vi "oa_SCL Min Max X.vi"(1 "scaled xy data":cluster{"x":i16, "y":i16}[](array[cluster])) -> (0 "min max data":cluster{"x":i16, "min":i16, "max":i16}[](array[cluster]))   [LabVIEW 2017]
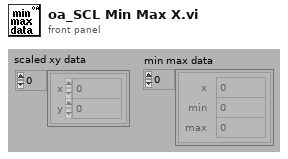
[diagram p1: front panel]
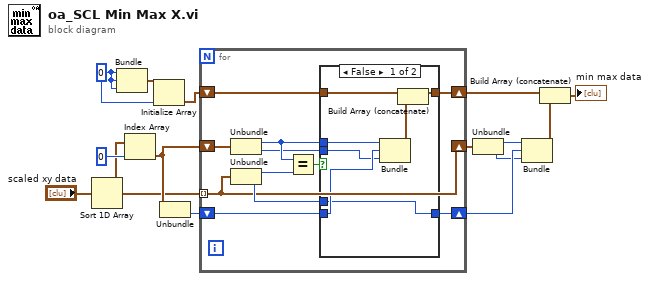
[diagram p0: block diagram]
diagram:
  w7 = i16 0
  n1 = Sort 1D Array(array="scaled xy data") -> (sorted array=w11:cluster{"x":i16, "y":i16}[])
  n2 = Bundle(w7, w7, w7) -> (w12:cluster{i16, i16, i16})  [unwired: 1 in]
  n3 = Index Array(array=w11, index=0) -> (element=w15:cluster{"x":i16, "y":i16})
  n4 = Initialize Array(w12, w7) -> (w13:cluster{i16, i16, i16}[])
  n5 = Unbundle(w15) -> ("y"=w5:i16)  [unwired: 1 out]
  n6 = for {
    shift-right: [w16] -> w10
    shift-left: w15 -> [w21]
    shift-right: [w22] -> w6
    shift-left: w5 -> [w23]
    tunnel: w11 -> [w16] mode=indexing
    shift-right: [w24] -> w9
    shift-left: w13 -> [w25]
    n7 = Unbundle(w21) -> ("x"=w18:i16, "y"=w17:i16)
    n8 = Unbundle(w16) -> ("x"=w20:i16, "y"=w19:i16)
    n9 = Equal?(x=w18, y=w20) -> (x = y?=w26:bool)
    n10 = case shown="False" w26 {
      tunnel: w25 -> [w33 w35]
      tunnel: [w32 w35] -> w24
      tunnel: w23 -> [w31 w34]
      tunnel: [w29 w34] -> w22
      tunnel: w19 -> [w29 _]
      tunnel: w18 -> [w28 _]
      tunnel: w17 -> [w27 _]
      frame False {
        n11 = Bundle("x"=w28, "y"=w31, "y"=w27) -> (w30:cluster{"x":i16, "y":i16, "y":i16})  [unwired: 1 in]
        n12 = Build Array (concatenate)(w33, w30) -> (w32:cluster{"x":i16, "y":i16, "y":i16}[])
      }
      frame True {
      }
    }
  }
  n13 = Unbundle(w10) -> ("x"=w3:i16, "y"=w2:i16)
  n14 = Bundle("x"=w3, "y"=w6, "y"=w2) -> (w4:cluster{"x":i16, "y":i16, "y":i16})  [unwired: 1 in]
  n15 = Build Array (concatenate)(w9, w4) -> (→"min max data":cluster{"x":i16, "y":i16, "y":i16}[])
